vi "task_updateFirmware.vi"() -> ()   [LabVIEW 2015]
uses:
  Framework/pdbm_test_route/UsrDefine/TaskFeedbackCmd.ctl
  Framework/pdbm_test_route/UsrDefine/TaskReqst.ctl
  <vilib>/DAQmx/read.llb/DAQmx Read (Analog Wfm 1Chan NSamp).vi
  <vilib>/Utility/file.llb/Write Delimited Spreadsheet (string).vi
  <vilib>/measure/matone.llb/Extract Multiple Tone Information 1 Chan.vi
  <vilib>/DAQmx/miscellaneous.llb/DAQmx Fill In Error Info.vi
  <vilib>/measure/madcrms.llb/Basic Averaged DC-RMS for 1 Chan.vi
  <vilib>/measure/matone.llb/Extract Single Tone Information 1 Chan.vi
  Framework/pdbm_tasks/pdbm_tasks.lvlib
  <vilib>/measure/NI_MAPro.lvlib
  <vilib>/measure/NI_MABase.lvlib
  Framework/pdbm_test_route/pdbm_task_route.lvlib
panel:
  in  "uA_bank0":dbl=1.5 format="%#_13g"
  out "Sample rate":dbl=20000.0 format="%#_13g"
  out "Ver":string
  out "Task out":refnum<k21>="Stop"
  in  "Tab Control":enum32{"Current Tracking", "Image", "CSV LOG"}(tab)
  out "uA_bank1":dbl
  in  "Calib":bool
  in  "Power ON/OFF":bool
  in  "Profile":enum16{"SAM", "DIANA", "Other..."}(ring)
  in  "Take Picture":bool
  in  "Orginal":bool
  in  "Clear Graph":bool
  out "Amp(Vdc)":dbl
  out "Freq(Hz)":dbl
  out "Waveform Graph 3":waveform(dbl)(graph)
  in  "ZOOM M1M2":bool
  in  "ZOOM -":bool
  in  "ZOOM +":bool
  in  "stop":bool
  out "VDUT- Vbat":dbl
  in  "Acquire Mode":enum16{"Streaming", "Read All", "Stop"}(ring)
  in  "Measure":bool
  in  "Current Range":T1(ring)
  out "Source":dbl
  in  "USB":tag="Dev1"
  out "Min value":dbl
  out "Max value":dbl
  out "Delta(s)":sgl
  in  "Center":bool
  out "Average":dbl
  in  "mA/uA":bool
  out "Waveform_main":waveform(sgl)(graph)
  out "Waveform_sub":waveform(dbl)(graph)
  out "Average (uA)":dbl
  in  "DUT Voltage Selector":enum16{"3.8VDC", "2.9VDC", "3.7VDC", "4.0VDC"}(ring)=enum."2.9VDC"
  in  "file List":i32(listbox)
  out "2D Picture":picture
  out "uA 2":dbl format="%#_4g"
  out "Vbat":dbl format="%#_4g"
  out "current time":timestamp
  in  "Record uA & Vbat":bool
  in  "Path":path
  out "uA":dbl(graph)
  out "Vbat Monitor":dbl(graph)
  out "error out":errorcluster
  out "seconds since 1Jan1904":timestamp
  out "new_ver":string caption="New Version :"
  out "curr_version":string caption="Current Version :"
  out "Clear":bool=TRUE
  in  "error in (no error)":errorcluster
  in  "pdbm_task_data":T2
  # "Current"
  # "Voltage"
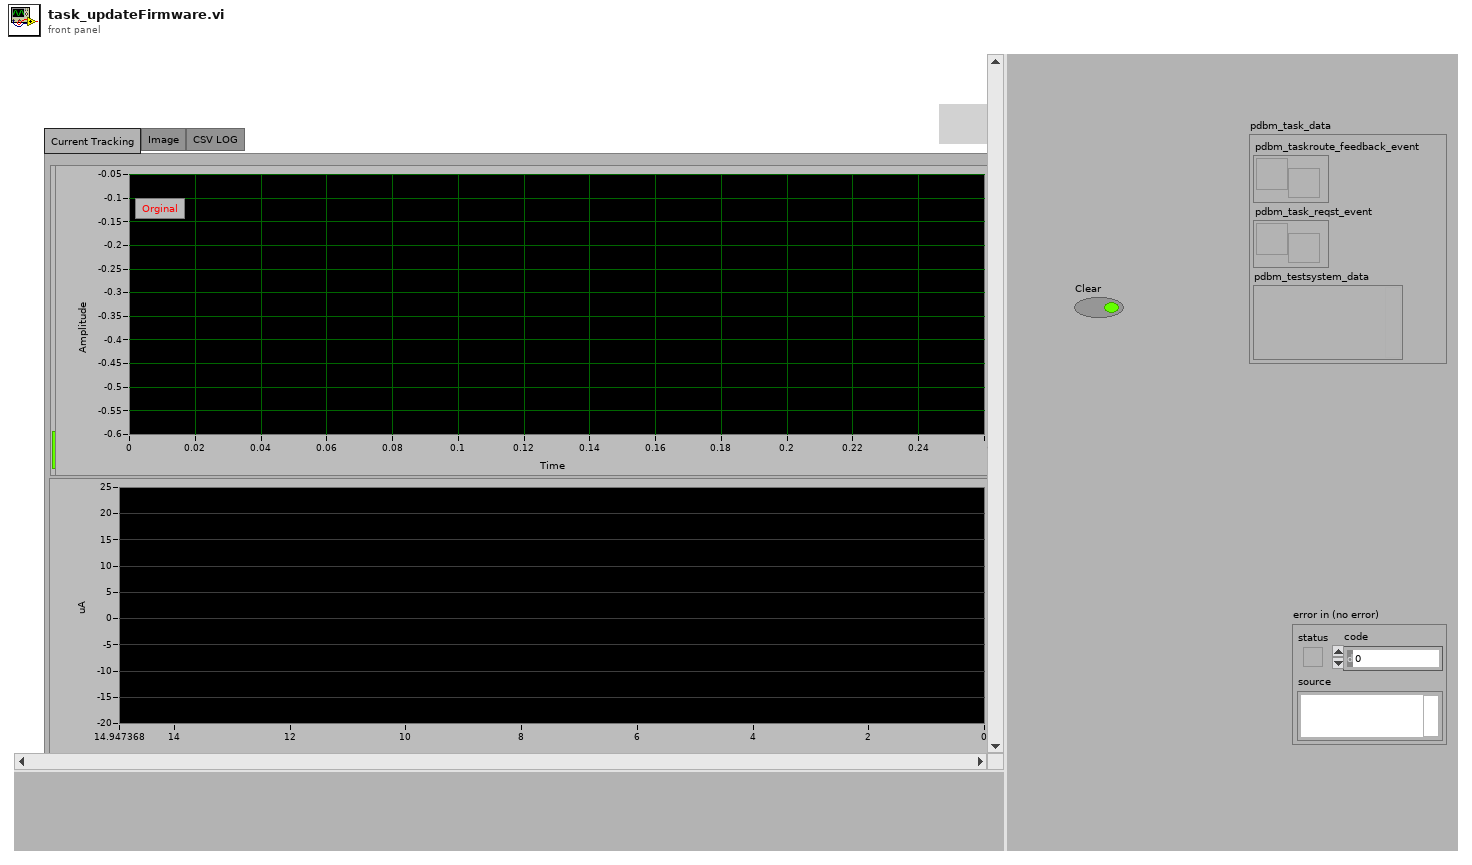
[diagram p1: front panel]
types:
  T1 = enum16{"Set uA Range ", "Set mA Range", "Measure Voltage"}
  T2 = cluster{"pdbm_taskroute_feedback_event":refnum<user-event>, "pdbm_task_reqst_event":refnum<user-event>, "pdbm_testsystem_data":variant}
  T3 = typedef "pdbm_tasks.lvlib/PDBM_TestSystem_Data.ctl" = cluster{"pdbm_general_report_info":refnum<vi>, "pdbm_task_progress":refnum<vi>, "pdbm_TestButton":refnum<vi>}
  T4 = cluster{"pdbm_task_reqst_event":refnum<user-event>, "pdbm_taskroute_feedback_event":refnum<user-event>}
  T5 = typedef "LVCursorListTypeDef.ctl" = cluster{"Name":string, "Color":u32, "Style":u8, "Point Style":u8, "Name Visible":bool, "Allow Drag":bool, "Cursor Mode":u32, "Plot":i32, "Index":i32, "Position":cluster{"X":dbl, "Y":dbl}, "X Scale":u32, "Y Scale":u32, "Watch Plots":i32[], "Watch All Plots":bool, "Plot Area":i32, "Label Offset":cluster{"X":dbl, "Y":dbl}}[]
  T6 = typedef "imagedata.ctl" = cluster{"image type":i32, "image depth":i32, "image":u8[], "mask":u8[], "colors":u32[], "Rectangle":cluster{"left":i16, "top":i16, "right":i16, "bottom":i16}}
  T7 = enum32{"none", "input signal", "detected signal", "residual signal"}
  T8 = cluster{"detected frequency":dbl, "detected amplitude":dbl, "detected phase (deg)":dbl}[]
  T9 = cluster{"detected frequency":dbl, "detected amplitude":dbl, "detected phase (deg)":dbl}
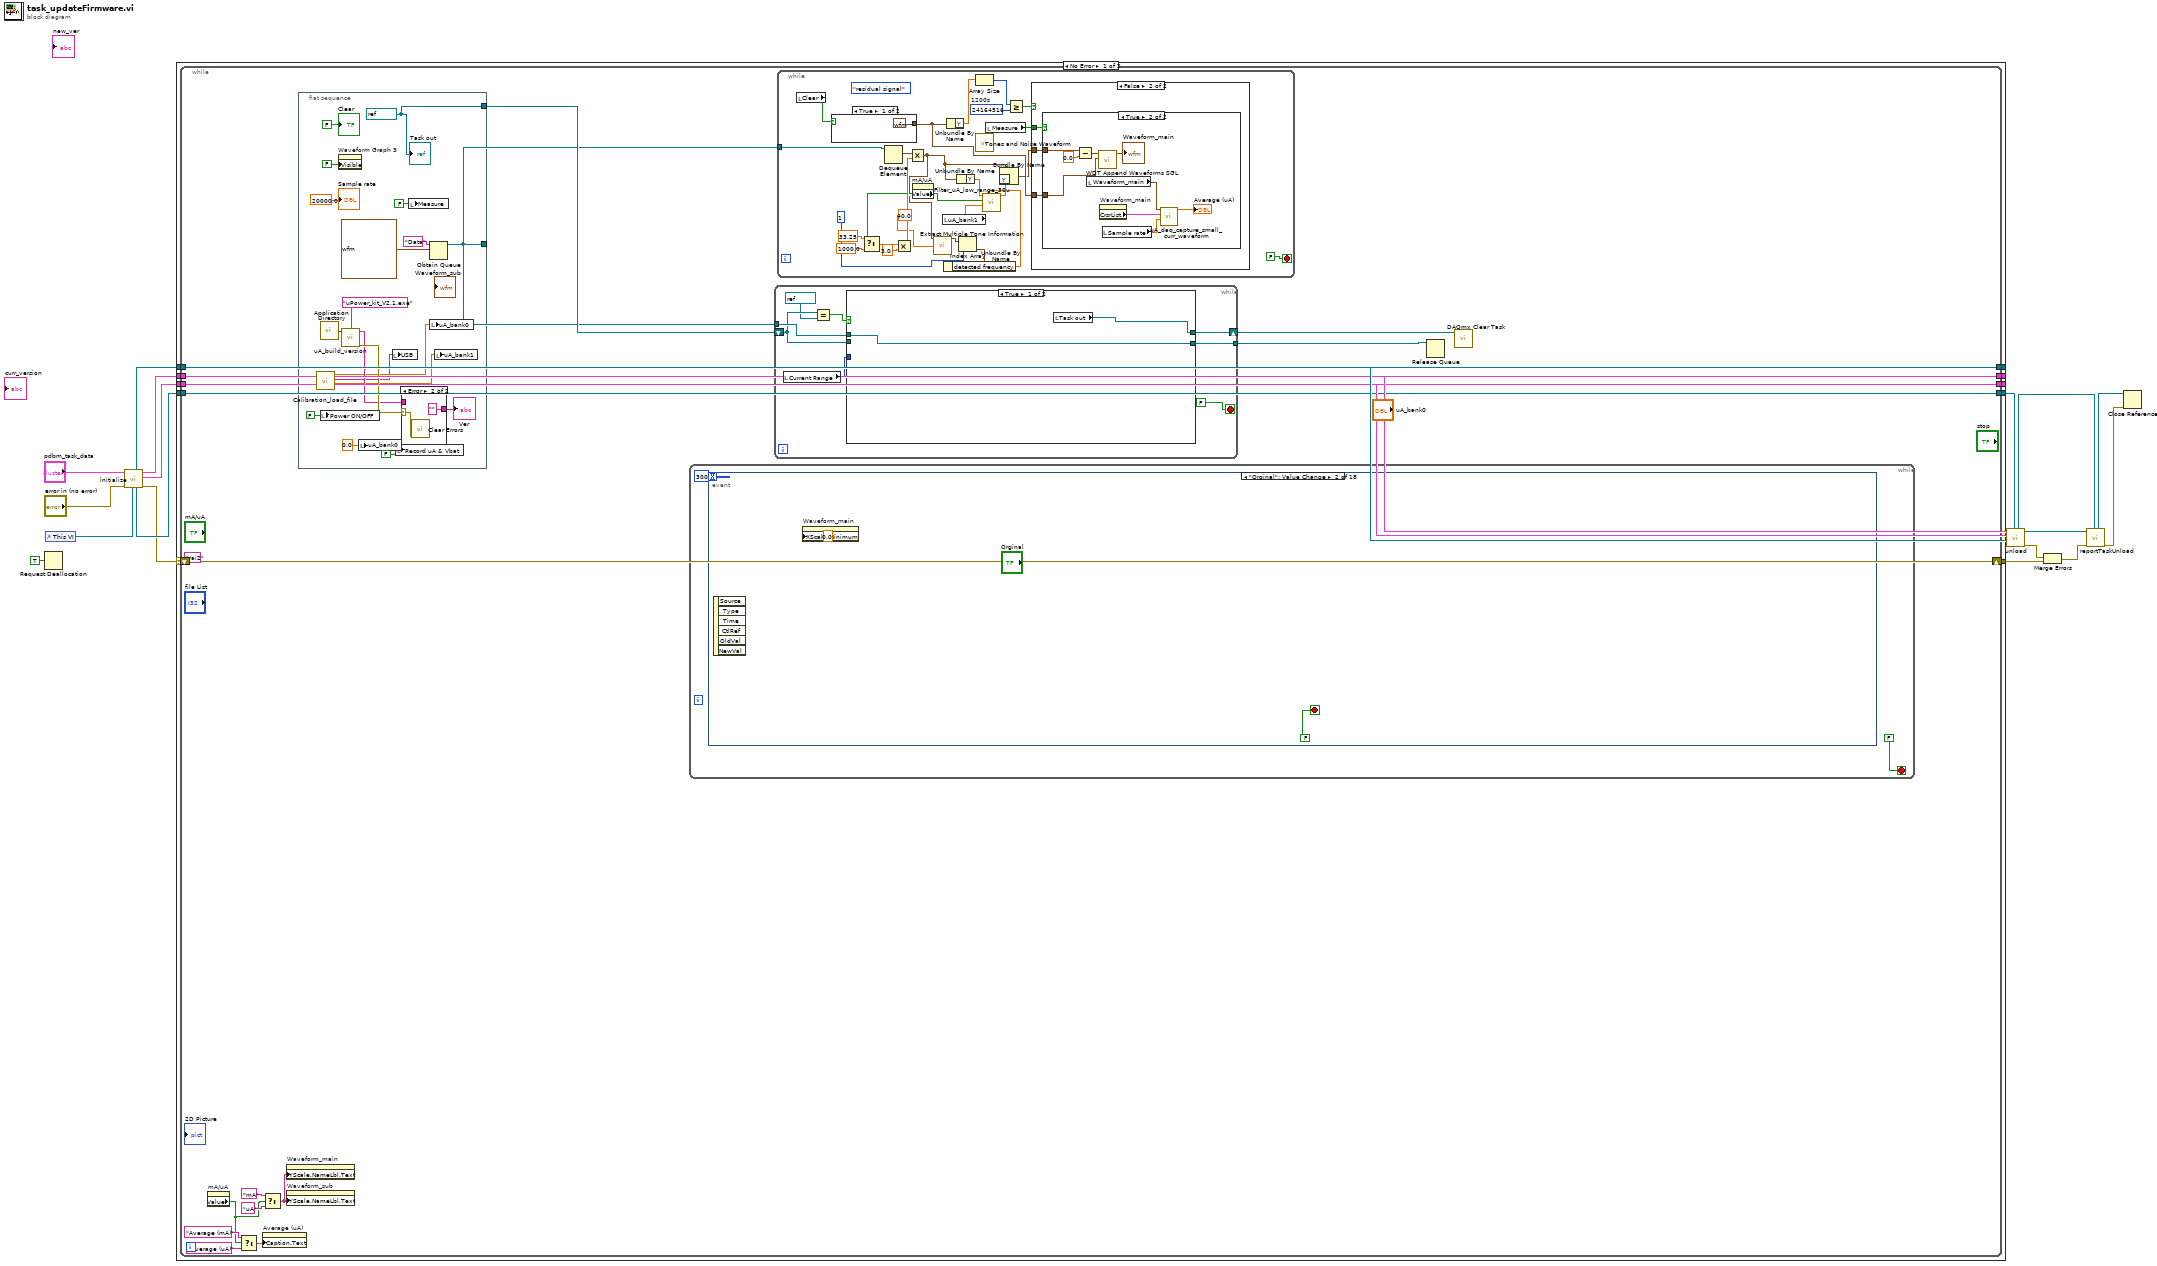
[diagram p0: block diagram]
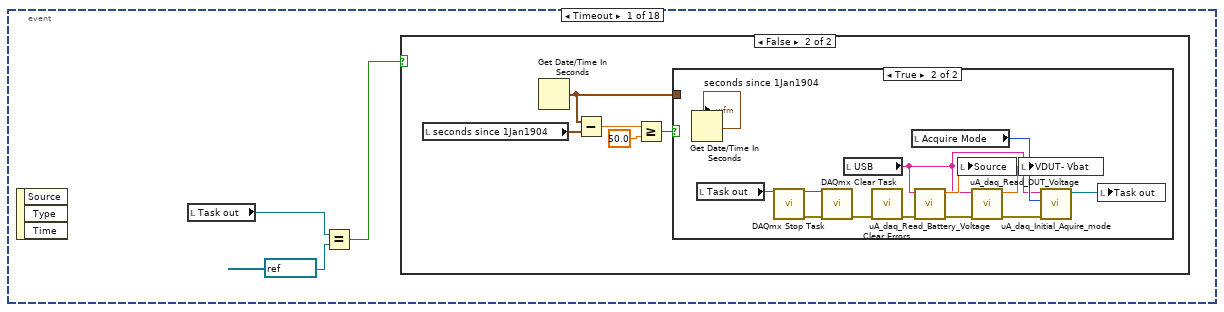
[diagram p3: hidden frame]
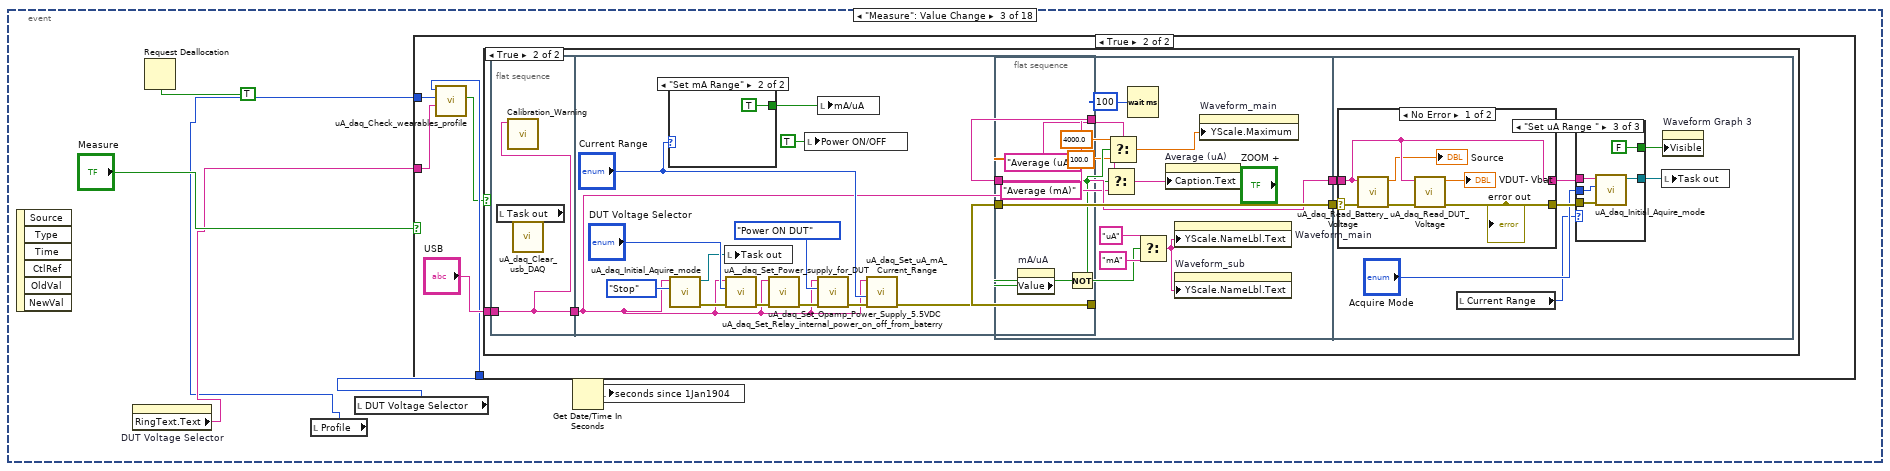
[diagram p6: hidden frame]
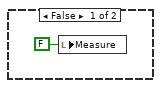
[diagram p8: hidden frame]
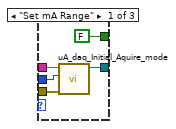
[diagram p9: hidden frame]
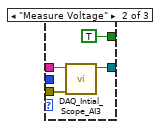
[diagram p10: hidden frame]
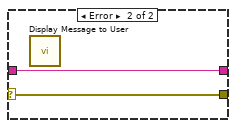
[diagram p11: hidden frame]
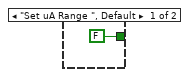
[diagram p12: hidden frame]
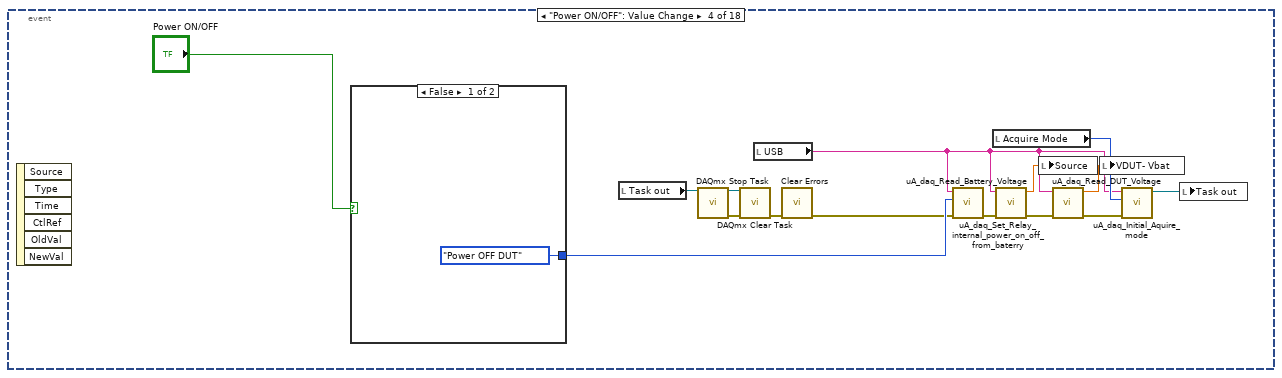
[diagram p13: hidden frame]
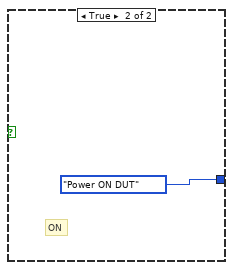
[diagram p14: hidden frame]
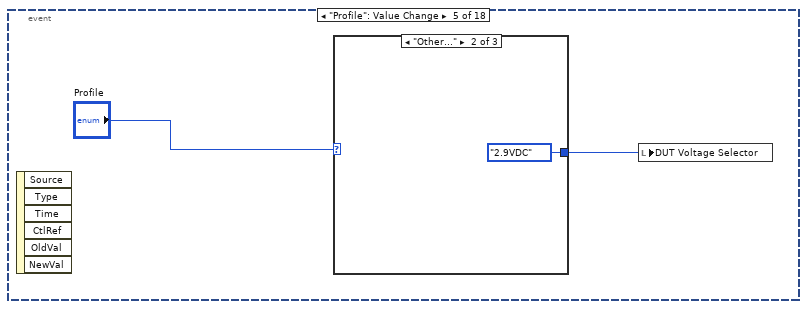
[diagram p15: hidden frame]
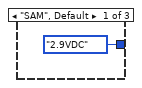
[diagram p16: hidden frame]
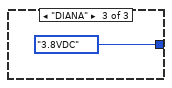
[diagram p17: hidden frame]
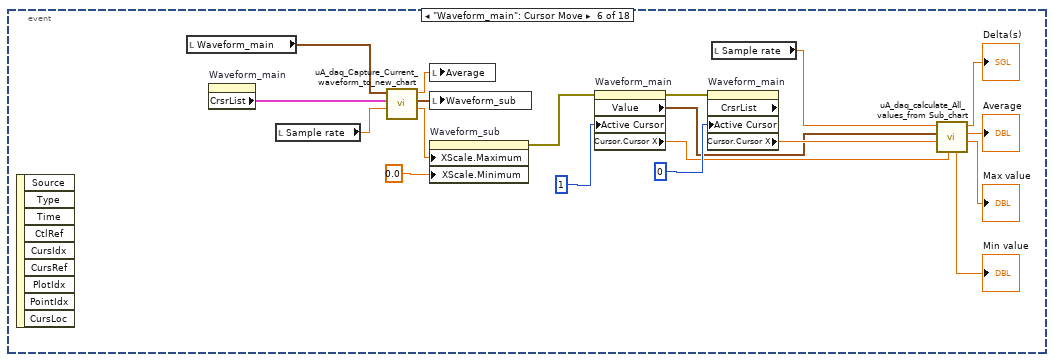
[diagram p18: hidden frame]
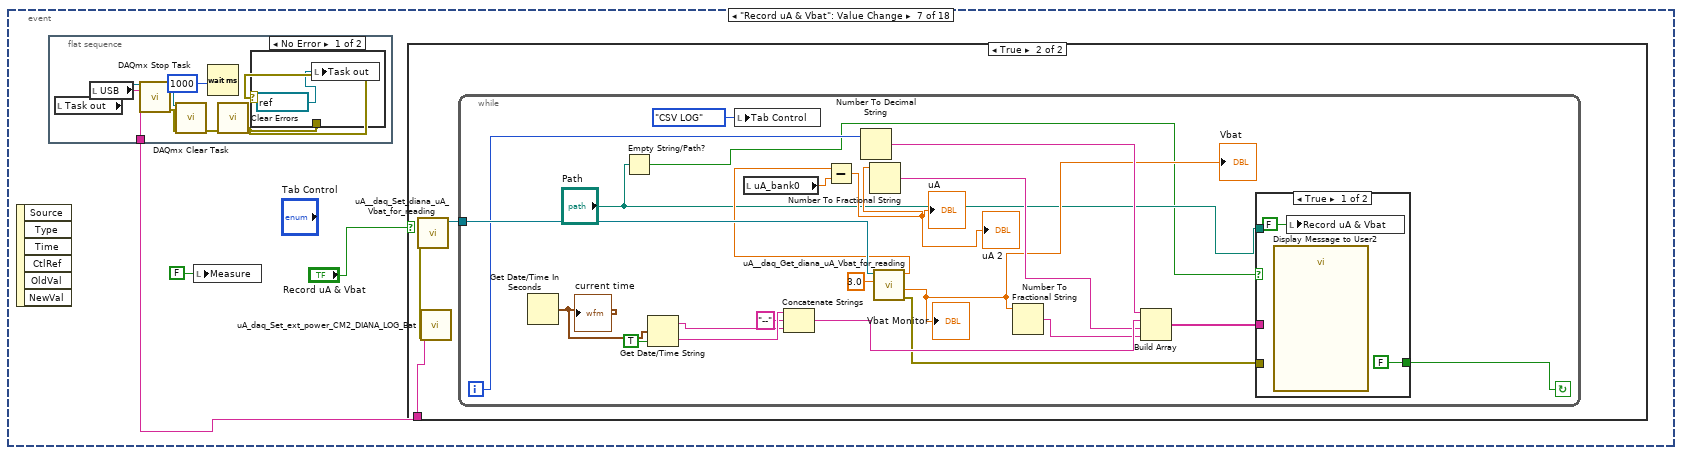
[diagram p19: hidden frame]
diagram:
  n1 = Request Deallocation(TRUE ("flag")) -> ()
  n2 = control-ref of="This VI"() -> (w19:refnum<vi>)
  n3 = call "initialize.vi"("TaskRef in"=w19, "error in"="error in (no error)", "pdbm_task_data"="pdbm_task_data") -> ("error out"=w15:errorcluster, "pdbm_task_data"=w3:T3, "pdbm_task_event"=w16:T4, "TaskRef out"=w17:refnum<vi>, "pdbm_task_reg_reqst_event"=w14:refnum<event-registration>)  [unwired: 4 in]
  n4 = case shown="No Error" w15 {
    selector: w15 -> [w29 w454]
    tunnel: w3 -> [w27 w452]
    tunnel: [w28 w454] -> w10
    tunnel: w17 -> [w22 w451]
    tunnel: w16 -> [w26 w453]
    tunnel: w14 -> [w30 w450]
    tunnel: [w25 w453] -> w13
    tunnel: [w24 w452] -> w12
    tunnel: [w23 w451] -> w2
    tunnel: [w21 w450] -> w11
    frame No Error {
      n5 = while {
        tunnel: w30 -> [w44]
        shift-right: [w43] -> w28
        shift-left: w29 -> [w43]
        tunnel: w22 -> [w45]
        tunnel: w27 -> [w46]
        tunnel: w26 -> [w47]
        tunnel: [w47] -> w25
        tunnel: [w46] -> w24
        tunnel: [w45] -> w23
        tunnel: [w44] -> w21
        stop <- FALSE ("stop") stop-if-true
        (unwired) "/ai2" ("string")
        n6 = property on="mA/uA" class="Bool (strict)"() -> ("Value"=w36:bool)  [unwired: 2 in, 2 out]
        n7 = Select(t="Average (mA)" ("Caption.Text"), s=w36, f="Average (uA)" ("Caption.Text")) -> (s? t:f=w34:string)
        n8 = property on="Average (uA)" class="DigNum (strict)"("Caption.Text"=w34) -> ()  [unwired: 2 in, 2 out]
        n9 = Select(t="mA" ("Caption.Text"), s=w36, f="uA" ("Caption.Text")) -> (s? t:f=w35:string)
        n10 = property on="Waveform_main" class="WFGraph (strict)"("YScale.NameLbl.Text"=w35) -> ()  [unwired: 2 in, 2 out]
        n11 = property on="Waveform_sub" class="WFGraph (strict)"("YScale.NameLbl.Text"=w35) -> ()  [unwired: 2 in, 2 out]
        n12 = flat-sequence {
          tunnel: [w58] -> w32
          tunnel: [w61] -> w31
          frame #0 {
            w58 = refnum<k21> "Stop" ("task out")
            n13 = call "Calibration_load_file.vi"() -> ("uABank1"=w51:dbl, "USB_DEV"=w50:string, "uABank0"=w52:dbl)  [unwired: 9 in]
            n14 = call <vilib>:"Application Directory.vi"() -> ("Application Directory"=w60:path)
            n15 = local write "Power ON/OFF"(FALSE ("Power ON/OFF")) -> ()
            n16 = property on="Waveform Graph 3" class="WFGraph (strict)"("Visible"=FALSE) -> ()  [unwired: 2 in, 2 out]
            n17 = call "uA_build_version.vi"("name or relative path"="uPower_kit_V2.1.exe", "path"=w60) -> ("error out"=w57:errorcluster, "FileVersion"=w56:string)  [unwired: 7 in, 1 out]
            n18 = local write "uA_bank0"(0.0 ("uA_calib_0")) -> ()
            n19 = local write "USB"(w50) -> ()
            n20 = local write "Record uA & Vbat"(FALSE ("Record uA & Vbat")) -> ()
            n21 = case shown="Error" w57 {
              selector: w57 -> [_ w69]
              tunnel: w56 -> [w67 _]
              tunnel: [w67 "" ("FileVersion")] -> w55
              frame No Error {
              }
              frame Error {
                n22 = call <vilib>:"Clear Errors.vi"("error in (no error)"=w69) -> ()  [unwired: 5 in, 2 out]
              }
            }
            "Ver" <- w55
            n23 = local write "Measure"(FALSE ("Measure")) -> ()
            n24 = Obtain Queue(name (unnamed)="Data", element data type=waveform(sgl) {"t0"=timestamp(0 s since 1904-01-01), "dt"=1.0, "Y"=[]} ("Waveform Chart 2")) -> (queue out=w61:refnum<queue>)  [unwired: 3 in, 2 out]
            n25 = local write "uA_bank0"(w52) -> ()
            n26 = local write "uA_bank1"(w51) -> ()
            "Clear" <- FALSE ("Clear")
            "Sample rate" <- 20000.0 ("Sample rate")
            "Task out" <- w58
          }
        }
        n27 = while {
          stop <- FALSE stop-if-true
          n28 = event shown="[1] \"Orginal\": Value Change" {
            selector: _ -> [_ _ _ _ _ _ _ _ _ _ _ _ _ _ _ _ _ _]
            dyn-events: _ -> [_ _ _ _ _ _ _ _ _ _ _ _ _ _ _ _ _ _]
            timeout: 300 -> [_ _ _ _ _ _ _ _ _ _ _ _ _ _ _ _ _ _]
            event Timeout {
              n29 = event-data() -> ()  [unwired: 1 in, 3 out]
              n30 = local read "Task out"() -> (w72:refnum<k21>)
              n31 = Equal?(x=w72, y=refnum<k21> "Stop") -> (x = y?=w73:bool)
              n32 = case shown="False" w73 {
                frame True {
                }
                frame False {
                  n33 = local read "seconds since 1Jan1904"() -> (w75:timestamp)
                  n34 = Get Date/Time In Seconds() -> (seconds since 1Jan1904=w76:timestamp)
                  n35 = Subtract(x=w76, y=w75) -> (x-y=w79:dbl)
                  n36 = Greater Or Equal?(x=w79, y=50.0) -> (x >= y?=w77:bool)
                  n37 = case shown="True" w77 {
                    tunnel: w76 -> [_ _]
                    frame False {
                    }
                    frame True {
                      n38 = Get Date/Time In Seconds() -> (seconds since 1Jan1904=→"seconds since 1Jan1904":timestamp)
                      n39 = local read "Task out"() -> (w89:refnum<k21>)
                      n40 = call <vilib>:"DAQmx Stop Task.vi"("task/channels in"=w89) -> ("task out"=w88:refnum<k21>, "error out"=w91:errorcluster)  [unwired: 13 in]
                      n41 = call <vilib>:"DAQmx Clear Task.vi"("task in"=w88, "error in"=w91) -> ("error out"=w90:errorcluster)  [unwired: 13 in]
                      n42 = local read "USB"() -> (w82:tag)
                      n43 = call <vilib>:"Clear Errors.vi"("error in (no error)"=w90) -> ("error out"=w87:errorcluster)  [unwired: 5 in, 1 out]
                      n44 = local read "Acquire Mode"() -> (w83:enum16{"Streaming", "Read All", "Stop"})
                      n45 = call "uA_daq_Read_Battery_Voltage.vi"("error in"=w87, "USB DAQ"=w82) -> ("error out"=w84:errorcluster, "Battery_Voltage"=w86:dbl)  [unwired: 8 in]
                      n46 = local write "Source"(w86) -> ()
                      n47 = call "uA_daq_Read_DUT_Voltage.vi"("error in"=w84, "USB DAQ"=w82) -> ("error out"=w81:errorcluster, "DUT_Voltage"=w85:dbl)  [unwired: 8 in]
                      n48 = local write "VDUT- Vbat"(w85) -> ()
                      n49 = call "uA_daq_Initial_Aquire_mode.vi"("error in"=w81, "Acquire Mode"=w83, "USB DAQ"=w82) -> ("Refnum out"=w80:refnum<k21>)  [unwired: 7 in, 1 out]
                      n50 = local write "Task out"(w80) -> ()
                    }
                  }
                }
              }
            }
            event "Orginal": Value Change {
              n51 = event-data() -> ()  [unwired: 1 in, 6 out]
              n52 = property on="Waveform_main" class="WFGraph (strict)"("XScale.Minimum"=0.0 ("X Scale.Range:Minimum")) -> ()  [unwired: 2 in, 2 out]
            }
            event "Measure": Value Change {
              n53 = event-data() -> ()  [unwired: 1 in, 6 out]
              n54 = property on="DUT Voltage Selector" class="Enum (strict)"() -> ("RingText.Text"=w96:string)  [unwired: 2 in, 2 out]
              n55 = Request Deallocation(TRUE ("flag")) -> ()
              n56 = local read "Profile"() -> (w94:enum16{"SAM", "DIANA", "Other..."})
              n57 = local read "DUT Voltage Selector"() -> (w95:enum16{"3.8VDC", "2.9VDC", "3.7VDC", "4.0VDC"})
              n58 = case shown="True" "Measure" {
                tunnel: w96 -> [_ w103]
                tunnel: w95 -> [_ w102]
                tunnel: w94 -> [_ w101]
                frame False {
                }
                frame True {
                  n59 = call "uA_daq_Check_wearables_profile.vi"("VDUT"=w103, "Profile"=w101, "DUT Voltage Selector"=w102) -> ("Profile"=w100:bool)  [unwired: 7 in, 1 out]
                  n60 = case shown="True" w100 {
                    tunnel: "USB" -> [_ w107]
                    frame False {
                      n61 = local write "Measure"(FALSE ("Measure")) -> ()
                    }
                    frame True {
                      n62 = flat-sequence {
                        tunnel: w107 -> [w156]
                        tunnel: [w156] -> w111
                        tunnel: [w165] -> w108
                        tunnel: [w159] -> w106
                        tunnel: w111 -> [w159]
                        frame #0 {
                          n63 = local read "Task out"() -> (w157:refnum<k21>)
                          n64 = call "Calibration_Warning.vi"("USB"=w156) -> ()  [unwired: 11 in]
                          n65 = call "uA_daq_Clear_usb_DAQ.vi"("Refnum in"=w157) -> ()  [unwired: 11 in]
                        }
                        frame #1 {
                          n66 = case shown="\"Set mA Range\"" "Current Range" {
                            tunnel: [FALSE ("mA/uA") TRUE ("mA/uA")] -> w163
                            frame "Set uA Range ", Default {
                            }
                            frame "Set mA Range" {
                            }
                          }
                          n67 = call "uA_daq_Initial_Aquire_mode.vi"("Acquire Mode"=enum16{"Streaming", "Read All", "Stop"}."Stop", "USB DAQ"=w159) -> ("error out"=w160:errorcluster, "Refnum out"=w161:refnum<k21>)  [unwired: 8 in]
                          n68 = local write "Task out"(w161) -> ()
                          n69 = call "uA__daq_Set_Power_supply_for_DUT.vi"("error in"=w160, "DUT Voltage Selector"="DUT Voltage Selector", "USB DAQ"=w159) -> ("error out"=w169:errorcluster)  [unwired: 8 in]
                          n70 = call "uA_daq_Set_Opamp_Power_Supply_5.5VDC.vi"("error in"=w169, "USB DAQ"=w159) -> ("error out"=w167:errorcluster)  [unwired: 9 in]
                          n71 = local write "Power ON/OFF"(TRUE ("Power ON/OFF")) -> ()
                          n72 = local write "mA/uA"(w163) -> ()
                          n73 = call "uA_daq_Set_Relay_internal_power_on_off_from_baterry.vi"("error in"=w167, "Power ON/OFF DUT"=enum16{"Power ON DUT", "Power OFF DUT"}."Power ON DUT", "USB DAQ"=w159) -> ("error out"=w166:errorcluster)  [unwired: 8 in]
                          n74 = call "uA_daq_Set_uA_mA_Current_Range.vi"("error in"=w166, "Current Range"="Current Range", "device name"=w159) -> ("error out"=w165:errorcluster)  [unwired: 8 in]
                        }
                      }
                      n75 = flat-sequence {
                        tunnel: w106 -> [w124]
                        tunnel: w108 -> [w125]
                        tunnel: [w125] -> w110
                        tunnel: [w124] -> w109
                        tunnel: w110 -> [w133]
                        tunnel: w109 -> [w132]
                        frame #0 {
                          n76 = property on="mA/uA" class="Bool (strict)"() -> ("Value"=w116:bool)  [unwired: 2 in, 2 out]
                          n77 = Not(x=w116) -> (.not. x?=w115:bool)
                          n78 = Select(t="Average (uA)" ("Caption.Text"), s=w115, f="Average (mA)" ("Caption.Text")) -> (s? t:f=w122:string)
                          n79 = Select(t=4000.0, s=w115, f=100.0) -> (s? t:f=w114:dbl)
                          n80 = Wait (ms)(milliseconds to wait=u32 100) -> ()  [unwired: 1 out]
                          n81 = Select(t="uA" ("Caption.Text"), s=w115, f="mA" ("Caption.Text")) -> (s? t:f=w117:string)
                          n82 = property on="Average (uA)" class="DigNum (strict)"("Caption.Text"=w122) -> ()  [unwired: 2 in, 2 out]
                          n83 = property on="Waveform_main" class="WFGraph (strict)"("YScale.NameLbl.Text"=w117) -> ()  [unwired: 2 in, 2 out]
                          n84 = property on="Waveform_sub" class="WFGraph (strict)"("YScale.NameLbl.Text"=w117) -> ()  [unwired: 2 in, 2 out]
                          n85 = property on="Waveform_main" class="WFGraph (strict)"("YScale.Maximum"=w114) -> ()  [unwired: 2 in, 2 out]
                        }
                        frame #1 {
                          n86 = case shown="No Error" w133 {
                            selector: w133 -> [w151 w155]
                            tunnel: w132 -> [w149 w154]
                            tunnel: [w150 w155] -> w131
                            tunnel: [w149 w154] -> w130
                            frame No Error {
                              n87 = call "uA_daq_Read_Battery_Voltage.vi"("error in"=w151, "USB DAQ"=w149) -> ("error out"=w153:errorcluster, "Battery_Voltage"=→"Source":dbl)  [unwired: 8 in]
                              n88 = call "uA_daq_Read_DUT_Voltage.vi"("error in"=w153, "USB DAQ"=w149) -> ("error out"=w150:errorcluster, "DUT_Voltage"=→"VDUT- Vbat":dbl)  [unwired: 8 in]
                              "error out" <- w150
                            }
                            frame Error {
                              n89 = call "Display Message to User"() -> ()  [unwired: 10 in, 2 out]
                            }
                          }
                          n90 = local read "Current Range"() -> (w127:T1)
                          n91 = case shown="\"Set uA Range \"" w127 {
                            tunnel: w131 -> [w138 w140 w147]
                            tunnel: w130 -> [w137 w142 w146]
                            tunnel: [w136 w141 w145] -> w129
                            tunnel: "Acquire Mode" -> [w135 _ w144]
                            tunnel: [FALSE ("Visible") TRUE ("Visible") FALSE ("Visible")] -> w126
                            frame "Set mA Range" {
                              n92 = call "uA_daq_Initial_Aquire_mode.vi"("error in"=w138, "Acquire Mode"=w135, "USB DAQ"=w137) -> ("Refnum out"=w136:refnum<k21>)  [unwired: 7 in, 1 out]
                            }
                            frame "Measure Voltage" {
                              n93 = call "DAQ_Intial_Scope_AI3.vi"("error in"=w140, "physical channel"=w142) -> ("task out"=w141:refnum<k21>)  [unwired: 8 in, 1 out]
                            }
                            frame "Set uA Range " {
                              n94 = call "uA_daq_Initial_Aquire_mode.vi"("error in"=w147, "Acquire Mode"=w144, "USB DAQ"=w146) -> ("Refnum out"=w145:refnum<k21>)  [unwired: 7 in, 1 out]
                            }
                          }
                          n95 = local write "Task out"(w129) -> ()
                          n96 = property on="Waveform Graph 3" class="WFGraph (strict)"("Visible"=w126) -> ()  [unwired: 2 in, 2 out]
                        }
                      }
                    }
                  }
                }
              }
              n97 = Get Date/Time In Seconds() -> (seconds since 1Jan1904=w98:timestamp)
              n98 = local write "seconds since 1Jan1904"(w98) -> ()
            }
            event "Power ON/OFF": Value Change {
              n99 = event-data() -> ()  [unwired: 1 in, 6 out]
              n100 = case shown="False" "Power ON/OFF" {
                tunnel: [enum16{"Power ON DUT", "Power OFF DUT"}."Power OFF DUT" ("Power ON/OFF DUT") enum16{"Power ON DUT", "Power OFF DUT"}."Power ON DUT" ("Power ON/OFF DUT")] -> w177
                frame False {
                }
                frame True {
                  # "ON"
                }
              }
              n101 = local read "Task out"() -> (w185:refnum<k21>)
              n102 = call <vilib>:"DAQmx Stop Task.vi"("task/channels in"=w185) -> ("task out"=w184:refnum<k21>, "error out"=w187:errorcluster)  [unwired: 13 in]
              n103 = call <vilib>:"DAQmx Clear Task.vi"("task in"=w184, "error in"=w187) -> ("error out"=w186:errorcluster)  [unwired: 13 in]
              n104 = local read "USB"() -> (w176:tag)
              n105 = call <vilib>:"Clear Errors.vi"("error in (no error)"=w186) -> ("error out"=w175:errorcluster)  [unwired: 5 in, 1 out]
              n106 = call "uA_daq_Set_Relay_internal_power_on_off_from_baterry.vi"("error in"=w175, "Power ON/OFF DUT"=w177, "USB DAQ"=w176) -> ("error out"=w174:errorcluster)  [unwired: 8 in]
              n107 = local read "Acquire Mode"() -> (w181:enum16{"Streaming", "Read All", "Stop"})
              n108 = call "uA_daq_Read_Battery_Voltage.vi"("error in"=w174, "USB DAQ"=w176) -> ("error out"=w173:errorcluster, "Battery_Voltage"=w183:dbl)  [unwired: 8 in]
              n109 = local write "Source"(w183) -> ()
              n110 = call "uA_daq_Read_DUT_Voltage.vi"("error in"=w173, "USB DAQ"=w176) -> ("error out"=w180:errorcluster, "DUT_Voltage"=w182:dbl)  [unwired: 8 in]
              n111 = local write "VDUT- Vbat"(w182) -> ()
              n112 = call "uA_daq_Initial_Aquire_mode.vi"("error in"=w180, "Acquire Mode"=w181, "USB DAQ"=w176) -> ("Refnum out"=w179:refnum<k21>)  [unwired: 7 in, 1 out]
              n113 = local write "Task out"(w179) -> ()
            }
            event "Profile": Value Change {
              n114 = event-data() -> ()  [unwired: 1 in, 6 out]
              n115 = case shown="\"Other...\"" "Profile" {
                tunnel: [enum16{"3.8VDC", "2.9VDC", "3.7VDC", "4.0VDC"}."2.9VDC" ("DUT Voltage Selector") enum16{"3.8VDC", "2.9VDC", "3.7VDC", "4.0VDC"}."2.9VDC" ("DUT Voltage Selector") enum16{"3.8VDC", "2.9VDC", "3.7VDC", "4.0VDC"}."3.8VDC" ("DUT Voltage Selector")] -> w190
                frame "SAM", Default {
                }
                frame "Other..." {
                }
                frame "DIANA" {
                }
              }
              n116 = local write "DUT Voltage Selector"(w190) -> ()
            }
            event "Waveform_main": Cursor Move {
              n117 = event-data() -> ()  [unwired: 1 in, 9 out]
              n118 = local read "Waveform_main"() -> (w203:waveform(sgl))
              n119 = property on="Waveform_main" class="WFGraph (strict)"() -> ("CrsrList"=w213:T5)  [unwired: 2 in, 2 out]
              n120 = local read "Sample rate"() -> (w202:dbl)
              n121 = call "uA_daq_Capture_Current_waveform_to_new_chart.vi"("Sample rate"=w202, "CrsrList"=w213, "Waveform_main"=w203) -> ("Numeric"=w210:dbl, "Waveform"=w211:waveform(sgl), "Numeric 2"=w212:sgl)  [unwired: 6 in]
              n122 = local write "Average"(w212) -> ()
              n123 = local write "Waveform_sub"(w211) -> ()
              n124 = property on="Waveform_sub" class="WFGraph (strict)"("XScale.Maximum"=w210, "XScale.Minimum"=0.0 ("X Scale.Range:Minimum")) -> (error out=w195:errorcluster)  [unwired: 2 in, 1 out]
              n125 = property on="Waveform_main" class="WFGraph (strict)"(error in=w195, "Active Cursor"=u32 1) -> (error out=w205:errorcluster, "Value"=w204:waveform(sgl), "Cursor.Cursor X"=w207:dbl)  [unwired: 1 in, 1 out]
              n126 = property on="Waveform_main" class="WFGraph (strict)" props=["CrsrList", "Active Cursor", "Cursor", "Cursor X"](error in=w205, "Active Cursor"=u32 0) -> ("Cursor.Cursor X"=w206:dbl)  [unwired: 1 in, 3 out]
              n127 = local read "Sample rate"() -> (w201:dbl)
              n128 = call "uA_daq_calculate_All_values_from Sub_chart.vi"("Cursor.Cursor X 2"=w207, "Cursor.Cursor X"=w206, "Value"=w204, "Sample rate"=w201) -> ("Max value"=→"Max value":dbl, "Average"=→"Average":dbl, "Delta(s)"=→"Delta(s)":sgl, "Min value"=→"Min value":dbl)  [unwired: 4 in]
            }
            event "Record uA & Vbat": Value Change {
              n129 = event-data() -> ()  [unwired: 1 in, 6 out]
              n130 = flat-sequence {
                tunnel: [w223] -> w215
                frame #0 {
                  n131 = local read "Task out"() -> (w219:refnum<k21>)
                  n132 = local read "USB"() -> (w223:tag)
                  n133 = call <vilib>:"DAQmx Stop Task.vi"("task/channels in"=w219) -> ("task out"=w218:refnum<k21>, "error out"=w221:errorcluster)  [unwired: 13 in]
                  n134 = call <vilib>:"DAQmx Clear Task.vi"("task in"=w218, "error in"=w221) -> ("error out"=w220:errorcluster)  [unwired: 13 in]
                  n135 = Wait (ms)(milliseconds to wait=u32 1000) -> ()  [unwired: 1 out]
                  n136 = call <vilib>:"Clear Errors.vi"("error in (no error)"=w220) -> ("error out"=w217:errorcluster)  [unwired: 5 in, 1 out]
                  n137 = case shown="No Error" w217 {
                    tunnel: w217 -> [_ _]
                    frame No Error {
                      n138 = local write "Task out"(refnum<k21> "Stop" ("y")) -> ()
                    }
                    frame Error {
                    }
                  }
                }
              }
              n139 = local write "Measure"(FALSE ("Measure")) -> ()
              n140 = case shown="True" "Record uA & Vbat" {
                tunnel: w215 -> [_ w227]
                frame False {
                }
                frame True {
                  n141 = call "uA_daq_Set_ext_power_CM2_DIANA_LOG_Bat.vi"("USB DAQ in"=w227) -> ("error out"=w228:errorcluster, "USB DAQ out"=w226:tag)  [unwired: 9 in]
                  n142 = call "uA__daq_Set_diana_uA_Vbat_for_reading.vi"("error in (no error)"=w228, "USB DAQ in"=w226) -> ("Refnum out"=w225:refnum<k21>)  [unwired: 8 in, 1 out]
                  n143 = while {
                    tunnel: w225 -> [w250]
                    i -> [w240]
                    stop <- w229 continue-if-true
                    n144 = Get Date/Time In Seconds() -> (seconds since 1Jan1904=w249:timestamp)
                    "current time" <- w249
                    n145 = Empty String/Path?(string/path="Path") -> (empty?=w230:bool)
                    n146 = Get Date/Time String(seconds (now)=w249, want seconds? (F)=TRUE) -> (date string=w247:string, time string=w248:string)  [unwired: 1 in]
                    n147 = local write "Tab Control"(enum32{"Current Tracking", "Image", "CSV LOG"}."CSV LOG" ("Tab Control")) -> ()
                    n148 = local read "uA_bank0"() -> (w235:dbl)
                    n149 = Concatenate Strings(w248, "--" ("string"), w247) -> (w245:string)
                    n150 = Number To Decimal String(number=w240) -> (decimal integer string=w239:string)  [unwired: 1 in]
                    n151 = call "uA__daq_Get_diana_uA_Vbat_for_reading.vi"("Coef"=3.0, "Refnum in"=w250) -> ("error out"=w236:errorcluster, "Vbat"=w238:dbl, "uA Current"=w234:dbl)  [unwired: 5 in, 2 out]
                    "Vbat Monitor" <- w238
                    "Vbat" <- w238
                    n152 = Subtract(x=w234, y=w235) -> (x-y=w233:dbl)
                    "uA" <- w233
                    "uA 2" <- w233
                    n153 = Number To Fractional String(number=w233) -> (F-format string=w244:string)  [unwired: 3 in]
                    n154 = Number To Fractional String(number=w238) -> (F-format string=w243:string)  [unwired: 3 in]
                    n155 = Build Array(w239, w245, w244, w243) -> (w242:string[])
                    n156 = case shown="True" w230 {
                      tunnel: w242 -> [_ w256]
                      tunnel: w236 -> [_ w255]
                      tunnel: "Path" -> [_ w254]
                      tunnel: [FALSE ("Record uA & Vbat") w253] -> w229
                      frame True {
                        n157 = call "Display Message to User2"() -> ()  [unwired: 10 in, 2 out]
                        n158 = local write "Record uA & Vbat"(FALSE ("Record uA & Vbat")) -> ()
                      }
                      frame False {
                        n159 = local read "Record uA & Vbat"() -> (w253:bool)
                        n160 = case shown="No Error" w255 {
                          tunnel: w256 -> [w260 _]
                          tunnel: w254 -> [w257 _]
                          frame No Error {
                            n161 = call-poly <vilib>:"Write Delimited Spreadsheet.vi"("file path (dialog if empty)"=w257, "1D data"=w260, "append to file? (F)"=TRUE, "delimiter (\\t)"=";" ("delimiter (\\t)")) -> ()  [unwired: 10 in, 2 out]
                          }
                          frame Error {
                          }
                        }
                      }
                    }
                  }
                }
              }
            }
            event "Calib": Value Change {
              n162 = event-data() -> ()  [unwired: 1 in, 6 out]
              n163 = property on="mA/uA" class="Bool (strict)"() -> ("Value"=w263:bool)  [unwired: 2 in, 2 out]
              n164 = case shown="False" w263 {
                tunnel: [w264 _] -> w261
                frame False {
                  w271 = 3.0  # Coef 10Ohm:3
                  # "uA"
                  n165 = flat-sequence {
                    tunnel: [w280] -> w269
                    frame #0 {
                      n166 = call "Display Message to User3"() -> ()  [unwired: 10 in, 2 out]
                      n167 = local write "Measure"(FALSE ("Measure")) -> ()
                    }
                    frame #1 {
                      n168 = local read "Task out"() -> (w277:refnum<k21>)
                      n169 = Wait (ms)(milliseconds to wait=u32 1000) -> ()  [unwired: 1 out]
                      n170 = call <vilib>:"DAQmx Stop Task.vi"("task/channels in"=w277) -> ("task out"=w276:refnum<k21>, "error out"=w278:errorcluster)  [unwired: 13 in]
                      n171 = call <vilib>:"DAQmx Clear Task.vi"("task in"=w276, "error in"=w278) -> ("error out"=w275:errorcluster)  [unwired: 13 in]
                      n172 = case shown="No Error" w275 {
                        frame No Error {
                          n173 = local write "Task out"(refnum<k21> "Stop" ("y")) -> ()
                        }
                        frame Error {
                        }
                      }
                      n174 = local read "USB"() -> (w280:tag)
                    }
                  }
                  n175 = call "uA_daq_Set_ext_power_CM2_DIANA_LOG_Bat.vi"("USB DAQ in"=w269) -> ("error out"=w266:errorcluster, "USB DAQ out"=w273:tag)  [unwired: 9 in]
                  n176 = call "uA__daq_Set_diana_uA_Vbat_for_reading.vi"("error in (no error)"=w266, "USB DAQ in"=w273) -> ("error out"=w267:errorcluster, "Refnum out"=w272:refnum<k21>)  [unwired: 8 in]
                  n177 = call "uA__daq_Get_diana_uA_Vbat_for_reading.vi"("error in (no error)"=w267, "Coef"=w271, "Refnum in"=w272) -> ("error out"=w268:errorcluster, "uA Current"=w270:dbl)  [unwired: 4 in, 3 out]
                  n178 = local write "uA_bank0"(w270) -> ()
                  n179 = call "Calibration_Read_streaming_3s.vi"("error in (no error)"=w268, "USB"=w269) -> ("error out"=w264:errorcluster, "uABank1"=w265:dbl)  [unwired: 8 in]
                  "uA_bank1" <- w265
                  n180 = call "Calibration_Save_file.vi"("USB_DEV"=w269, "uABank1"=w265, "uABank0"=w270) -> ()  [unwired: 9 in]
                }
                frame True {
                  # "mA"
                }
              }
              n181 = call "Display Message to User4"("error in (no error)"=w261, "Enable"=TRUE) -> ()  [unwired: 8 in, 2 out]
            }
            event "Clear Graph": Value Change {
              n182 = event-data() -> ()  [unwired: 1 in, 6 out]
              n183 = flat-sequence {
                frame #0 {
                  w282 = waveform(sgl) {"t0"=timestamp(0 s since 1904-01-01), "dt"=1.0, "Y"=[]} ("Waveform_main")
                  n184 = local write "Waveform_main"(w282) -> ()
                  n185 = local write "Clear"(TRUE ("Clear")) -> ()
                  n186 = Wait (ms)(milliseconds to wait=u32 500) -> ()  [unwired: 1 out]
                  n187 = local write "Waveform_sub"(w282) -> ()
                }
                frame #1 {
                  n188 = local write "Clear"(FALSE ("Clear")) -> ()
                }
              }
            }
            event "ZOOM +": Value Change {
              n189 = event-data() -> ()  [unwired: 1 in, 6 out]
              n190 = property on="Waveform_main" class="WFGraph (strict)" props=["XScale", "Range", "XScale", "Increment", "XScale", "Maximum", "XScale", "Minimum"]() -> ("XScale.Maximum"=w291:dbl, "XScale.Minimum"=w287:dbl)  [unwired: 2 in, 4 out]
              n191 = Subtract(x=w291, y=0.1) -> (x-y=w289:dbl)
              n192 = Add(x=w287, y=0.1) -> (x+y=w286:dbl)
              n193 = property on="Waveform_main" class="WFGraph (strict)"("XScale.Maximum"=w289, "XScale.Minimum"=w286) -> ()  [unwired: 2 in, 2 out]
            }
            event "ZOOM -": Value Change {
              n194 = event-data() -> ()  [unwired: 1 in, 6 out]
              n195 = property on="Waveform_main" class="WFGraph (strict)" props=["XScale", "Range", "XScale", "Increment", "XScale", "Maximum", "XScale", "Minimum"]() -> ("XScale.Maximum"=w300:dbl, "XScale.Minimum"=w296:dbl)  [unwired: 2 in, 4 out]
              n196 = Subtract(x=w296, y=0.1) -> (x-y=w293:dbl)
              n197 = Less Than 0?(x=w293) -> (x < 0?=w295:bool)
              n198 = Add(x=w300, y=0.1) -> (x+y=w298:dbl)
              n199 = Select(t=0.0, s=w295, f=w293) -> (s? t:f=w292:dbl)
              n200 = property on="Waveform_main" class="WFGraph (strict)"("XScale.Maximum"=w298, "XScale.Minimum"=w292) -> ()  [unwired: 2 in, 2 out]
            }
            event "ZOOM M1M2": Value Change {
              n201 = event-data() -> ()  [unwired: 1 in, 6 out]
              n202 = property on="Waveform_main" class="WFGraph (strict)"("Active Cursor"=u32 0) -> (error out=w307:errorcluster)  [unwired: 2 in, 1 out]
              n203 = property on="Waveform_main" class="WFGraph (strict)"(error in=w307) -> (error out=w304:errorcluster, "Cursor.Cursor X"=w302:dbl)  [unwired: 1 in, 1 out]
              n204 = property on="Waveform_main" class="WFGraph (strict)"(error in=w304, "Active Cursor"=u32 1) -> (error out=w306:errorcluster)  [unwired: 1 in, 1 out]
              n205 = property on="Waveform_main" class="WFGraph (strict)"(error in=w306) -> ("Cursor.Cursor X"=w301:dbl)  [unwired: 1 in, 2 out]
              n206 = Greater?(x=w302, y=w301) -> (0:w303:bool)
              n207 = case shown="True" w303 {
                tunnel: w302 -> [w310 w312]
                tunnel: w301 -> [w309 w311]
                frame False {
                  n208 = property on="Waveform_main" class="WFGraph (strict)"("XScale.Maximum"=w309, "XScale.Minimum"=w310) -> ()  [unwired: 2 in, 2 out]
                }
                frame True {
                  n209 = property on="Waveform_main" class="WFGraph (strict)"("XScale.Maximum"=w312, "XScale.Minimum"=w311) -> ()  [unwired: 2 in, 2 out]
                }
              }
            }
            event "Waveform_main": Mouse Down {
              n210 = event-data() -> ()  [unwired: 1 in, 8 out]
            }
            event "Tab Control": Value Change {
              n211 = event-data() -> ()  [unwired: 1 in, 6 out]
              n212 = call <vilib>:"Application Directory.vi"() -> ("Application Directory"=w315:path)
              n213 = call <userlib>:"List Directory__ogtk.vi"("pattern"="*.bmp", "directory path"=w315) -> ("file names"=w313:string[])  [unwired: 2 in, 3 out]
              n214 = property on="file List" class="LstBox (strict)"("Item Names"=w313) -> ()  [unwired: 2 in, 2 out]
            }
            event "Center": Value Change {
              n215 = event-data() -> ()  [unwired: 1 in, 6 out]
              n216 = property on="Waveform_main" class="WFGraph (strict)"() -> ("XScale.Maximum"=w320:dbl, "XScale.Minimum"=w319:dbl)  [unwired: 2 in, 2 out]
              n217 = Add(x=w320, y=w319) -> (x+y=w318:dbl)
              n218 = Divide(x=w318, y=2.0) -> (x/y=w316:dbl)
              n219 = property on="Waveform_main" class="WFGraph (strict)" props=["Value", "Active Cursor", "Cursor", "Cursor X"]("Active Cursor"=u32 1, "Cursor.Cursor X"=w316) -> (error out=w321:errorcluster)  [unwired: 2 in, 2 out]
              n220 = property on="Waveform_main" class="WFGraph (strict)" props=["CrsrList", "Active Cursor", "Cursor", "Cursor X"](error in=w321, "Active Cursor"=u32 0, "Cursor.Cursor X"=w316) -> ()  [unwired: 1 in, 3 out]
            }
            event "stop": Value Change {
              n221 = event-data() -> ()  [unwired: 1 in, 6 out]
              n222 = flat-sequence {
                frame #0 {
                  n223 = local read "Task out"() -> (w325:refnum<k21>)
                  n224 = call <vilib>:"DAQmx Stop Task.vi"("task/channels in"=w325) -> ("task out"=w324:refnum<k21>, "error out"=w327:errorcluster)  [unwired: 13 in]
                  n225 = call <vilib>:"DAQmx Clear Task.vi"("task in"=w324, "error in"=w327) -> ("error out"=w326:errorcluster)  [unwired: 13 in]
                  n226 = call <vilib>:"Clear Errors.vi"("error in (no error)"=w326) -> ()  [unwired: 5 in, 2 out]
                }
                frame #1 {
                  n227 = local read "USB"() -> (w331:tag)
                  n228 = call "uA_daq_Set_Relay_internal_power_on_off_from_baterry.vi"("Power ON/OFF DUT"=enum16{"Power ON DUT", "Power OFF DUT"}."Power OFF DUT", "USB DAQ"=w331) -> ("error out"=w330:errorcluster)  [unwired: 9 in]
                  n229 = call "uA_daq_Set_Opamp_Power_Supply_Zero_voltageVDC.vi"("error in"=w330, "USB DAQ"=w331) -> ("error out"=w328:errorcluster)  [unwired: 9 in]
                  n230 = call <vilib>:"Clear Errors.vi"("error in (no error)"=w328) -> ()  [unwired: 5 in, 2 out]
                }
                frame #2 {
                  n231 = local read "Ver"() -> (w332:string)
                  n232 = Empty String/Path?(string/path=w332) -> (empty?=w333:bool)
                  n233 = case shown="True" w333 {
                    frame True {
                    }
                    frame False {
                      n234 = Quit LabVIEW(quit? (T)=TRUE) -> ()
                    }
                  }
                }
                frame #3 {
                  n235 = Stop(stop? (T)=TRUE) -> ()
                }
              }
            }
            event "file List": Value Change {
              n236 = event-data() -> ()  [unwired: 1 in, 6 out]
              n237 = property on="file List" class="LstBox (strict)"() -> ("Value"=w342:i32, "Item Names"=w343:string[])  [unwired: 2 in, 2 out]
              n238 = Index Array(array=w343, index=w342) -> (element=w338:string)
              n239 = call <vilib>:"Application Directory.vi"() -> ("Application Directory"=w339:path)
              n240 = Build Path(base path=w339, name or relative path=w338) -> (appended path=w337:path)
              n241 = call <vilib>:"Read BMP File.vi"("path to BMP file"=w337) -> ("image data"=w341:T6)  [unwired: 8 in, 2 out]
              n242 = call <vilib>:"Draw Flattened Pixmap.vi"("image data"=w341) -> ("new picture"=w340:picture)  [unwired: 8 in]
              n243 = property on="2D Picture" class="Pict"("Value"=w340, "ZoomFactor"=sgl 0.75 ("Zoom Factor")) -> ()  [unwired: 2 in, 2 out]
            }
            event "Take Picture": Value Change {
              n244 = event-data() -> ()  [unwired: 1 in, 6 out]
              n245 = call <vilib>:"Application Directory.vi"() -> ("Application Directory"=w345:path)
              n246 = call "File Dialog"("start path"=w345, "pattern (all files)"="*.bmp", "pattern label"="*.bmp") -> ("selected path"=w351:path, "error out"=w348:errorcluster)  [unwired: 9 in, 2 out]
              n247 = control-ref of="This VI"() -> (w349:refnum<vi>)
              n248 = invoke on="Invoke Node" class="VI" method="FP.Get Image"(reference=w349, "image depth"=enum32{"File", "Clipboard"}."File" ("Target")) -> ("image data"=w350:T6)  [unwired: 4 in, 5 out]
              n249 = call <vilib>:"Clear Errors.vi"("error in (no error)"=w348) -> ()  [unwired: 5 in, 2 out]
              n250 = call <vilib>:"Write BMP File.vi"("image data"=w350, "path to BMP file"=w351) -> ()  [unwired: 8 in, 2 out]
            }
          }
        }
        n251 = while {
          tunnel: w31 -> [w400]
          tunnel: [w399] -> w41
          shift-right: [w395] -> w33
          shift-left: w32 -> [w397]
          stop <- FALSE ("stop (F)") stop-if-true
          n252 = local read "Current Range"() -> (w394:T1)
          n253 = Equal?(x=w397, y=refnum<k21> "Stop") -> (x = y?=w393:bool)
          n254 = case shown="True" w393 {
            tunnel: w400 -> [w402 w407]
            tunnel: [w402 w406] -> w399
            tunnel: w397 -> [_ w405]
            tunnel: [w401 w404] -> w395
            tunnel: w394 -> [_ w403]
            frame True {
              n255 = local read "Task out"() -> (w401:refnum<k21>)
            }
            frame False {
              n256 = case shown="\"Set uA Range \"" w403 {
                tunnel: w407 -> [w418 w423 w445]
                tunnel: [w417 w423 w444] -> w406
                tunnel: w405 -> [w416 w434 w443]
                tunnel: [w415 w433 w442] -> w404
                frame "Set mA Range" {
                  w414 = 10.0  # timeout (s)
                  n257 = call-poly <vilib>:"DAQmx Read.vi"("task/channels in"=w416, "number of samples per channel"=10000, "timeout"=w414) -> ("data"=w409:waveform(dbl), "error out"=w412:errorcluster)  [unwired: 10 in, 1 out]
                  n258 = Unbundle By Name(w409) -> ("Y"=w411:dbl[])
                  n259 = Reverse 1D Array(array=w411) -> (reversed array=w408:dbl[])
                  n260 = Bundle By Name(cluster=w409, "Y"=w408) -> (w410:waveform(dbl))
                  n261 = case shown="No Error" w412 {
                    selector: w412 -> [_ w422]
                    tunnel: w418 -> [w421 _]
                    tunnel: [w420 _] -> w417
                    tunnel: w410 -> [w419 _]
                    frame No Error {
                      n262 = Enqueue Element(queue=w421, element=w419) -> (queue out=w420:refnum<queue>)  [unwired: 2 in, 2 out]
                    }
                    frame Error {
                      n263 = call <vilib>:"Clear Errors.vi"("error in (no error)"=w422) -> ()  [unwired: 5 in, 2 out]
                    }
                  }
                  n264 = local read "Task out"() -> (w415:refnum<k21>)
                }
                frame "Measure Voltage" {
                  w432 = 10.0  # timeout (s)
                  n265 = call-poly <vilib>:"DAQmx Read.vi"("task/channels in"=w434, "number of samples per channel"=5000, "timeout"=w432) -> ("data"=w427:waveform(dbl), "error out"=w430:errorcluster)  [unwired: 10 in, 1 out]
                  "Waveform Graph 3" <- w427
                  n266 = call <vilib>:"Clear Errors.vi"("error in (no error)"=w430) -> ()  [unwired: 5 in, 2 out]
                  n267 = call-poly <vilib>:"Basic Averaged DC-RMS.vi"("averaging type"=enum16{"Linear", "Exponential"}."Linear", "signal in"=w427) -> ("error out"=w424:errorcluster, "DC value"=→"Amp(Vdc)":dbl)  [unwired: 6 in, 2 out]
                  n268 = call-poly <vilib>:"Extract Single Tone Information.vi"("time signal in"=w427) -> ("error out"=w428:errorcluster, "detected frequency"=→"Freq(Hz)":dbl)  [unwired: 5 in, 4 out]
                  n269 = local read "Task out"() -> (w433:refnum<k21>)
                  n270 = call <vilib>:"Clear Errors.vi"("error in (no error)"=w428) -> ()  [unwired: 5 in, 2 out]
                  n271 = call <vilib>:"Clear Errors.vi"("error in (no error)"=w424) -> ()  [unwired: 5 in, 2 out]
                }
                frame "Set uA Range " {
                  w441 = 10.0  # timeout (s)
                  n272 = call-poly <vilib>:"DAQmx Read.vi"("task/channels in"=w443, "number of samples per channel"=10000, "timeout"=w441) -> ("data"=w436:waveform(dbl), "error out"=w439:errorcluster)  [unwired: 10 in, 1 out]
                  n273 = Unbundle By Name(w436) -> ("Y"=w438:dbl[])
                  n274 = Reverse 1D Array(array=w438) -> (reversed array=w435:dbl[])
                  n275 = Bundle By Name(cluster=w436, "Y"=w435) -> (w437:waveform(dbl))
                  n276 = case shown="Error" w439 {
                    selector: w439 -> [_ w449]
                    tunnel: w445 -> [w448 _]
                    tunnel: [w447 _] -> w444
                    tunnel: w437 -> [w446 _]
                    frame No Error {
                      n277 = Enqueue Element(queue=w448, element=w446) -> (queue out=w447:refnum<queue>)  [unwired: 2 in, 2 out]
                    }
                    frame Error {
                      n278 = call <vilib>:"Clear Errors.vi"("error in (no error)"=w449) -> ()  [unwired: 5 in, 2 out]
                    }
                  }
                  n279 = local read "Task out"() -> (w442:refnum<k21>)
                }
              }
            }
          }
        }
        n280 = while {
          tunnel: w31 -> [w373]
          stop <- FALSE stop-if-true
          (unwired) T7."residual signal" ("export mode")
          w366 = 24164516  # 1200s
          n281 = local read "Clear"() -> (w371:bool)
          n282 = case shown="True" w371 {
            tunnel: [waveform(sgl) {"t0"=timestamp(0 s since 1904-01-01), "dt"=1.0, "Y"=[]} ("Waveform_main") w392] -> w370
            frame True {
            }
            frame False {
              n283 = local read "Waveform_main"() -> (w392:waveform(sgl))
            }
          }
          n284 = Dequeue Element(queue=w373) -> (element=w372:waveform(sgl))  [unwired: 2 in, 3 out]
          n285 = property on="mA/uA" class="Bool (strict)"() -> ("Value"=w359:bool)  [unwired: 2 in, 2 out]
          n286 = Select(t=sgl 33.25 ("y"), s=w359, f=sgl 1000.0 ("y")) -> (s? t:f=w365:sgl)
          n287 = Multiply(x=w365, y=sgl 3.0) -> (x*y=w364:sgl)
          n288 = Multiply(x=w372, y=w364) -> (x*y=w357:waveform(sgl))
          n289 = call-poly <vilib>:"Extract Multiple Tone Information.vi"("time signal in"=w357, "threshold"=40.0 ("Numeric 2")) -> ("multiple tone information"=w356:T8)  [unwired: 11 in, 2 out]
          n290 = local read "uA_bank1"() -> (w358:dbl)
          n291 = Unbundle By Name(w370) -> ("Y"=w369:sgl[])
          n292 = Unbundle By Name(w357) -> ("Y"=w361:sgl[])
          n293 = Index Array(array=w356, index=u16 1 ("Index")) -> (element=w355:T9)
          n294 = Unbundle By Name(w355) -> ("detected frequency"=w352:dbl)
          n295 = Array Size(array=w369) -> (size(s)=w376:i32)
          n296 = call <vilib>:"Tones and Noise Waveform.vi"() -> ()  [unwired: 10 in, 2 out]
          n297 = call "Filter_uA_low_range_30u.vi"("Frequency"=w352, "uA_calib_0"=w358, "mA/uA"=w359, "in"=w361) -> ("out"=w360:dbl[])  [unwired: 7 in]
          n298 = local read "Measure"() -> (w368:bool)
          n299 = Bundle By Name(cluster=w357, "Y"=w360) -> (w362:waveform(sgl))
          n300 = Greater Or Equal?(x=w376, y=w366) -> (x >= y?=w367:bool)
          n301 = case shown="False" w367 {
            tunnel: w362 -> [_ w381]
            tunnel: w370 -> [_ w380]
            tunnel: w368 -> [_ w379]
            frame True {
              n302 = local write "Measure"(FALSE ("Measure")) -> ()
            }
            frame False {
              n303 = case shown="True" w379 {
                tunnel: w381 -> [_ w389]
                tunnel: w380 -> [_ w382]
                frame False {
                }
                frame True {
                  n304 = Subtract(x=w389, y=sgl 0.0) -> (x-y=w383:waveform(sgl))
                  n305 = local read "Waveform_main"() -> (w386:waveform(sgl))
                  n306 = call "WDT Append Waveforms SGL.vi"("waveform B"=w382, "waveform A"=w383) -> ("waveform out"=→"Waveform_main":waveform(sgl))  [unwired: 8 in, 1 out]
                  n307 = property on="Waveform_main" class="WFGraph (strict)"() -> ("CrsrList"=w387:T5)  [unwired: 2 in, 2 out]
                  n308 = local read "Sample rate"() -> (w385:dbl)
                  n309 = call "uA_daq_capture_small_curr_waveform.vi"("Sample rate"=w385, "CrsrList"=w387, "Waveform_main"=w386) -> ("Numeric"=→"Average (uA)":sgl)  [unwired: 8 in]
                }
              }
            }
          }
        }
        n310 = Release Queue(queue=w41) -> ()  [unwired: 2 in, 3 out]
        n311 = call <vilib>:"DAQmx Clear Task.vi"("task in"=w33) -> ()  [unwired: 14 in, 1 out]
      }
    }
    frame Error {
    }
  }
  n312 = call "unload.vi"("TaskRef in"=w2, "pdbm_task_reg_reqst_event"=w11, "pdbm_task_data"=w12, "pdbm_task_event"=w13) -> ("error out"=w9:errorcluster, "pdbm_taskroute_feedback_event"=w8:refnum<user-event>, "TaskRef out"=w1:refnum<vi>)  [unwired: 5 in]
  n313 = Merge Errors(w9, w10) -> (w7:errorcluster)
  n314 = call "reportTaskUnload.vi"("TaskRef"=w1, "error in (no error)"=w7, "pdbm_taskroute_feedback_event"=w8) -> ("error out"=w4:errorcluster, "TaskRef out"=w5:refnum<vi>)  [unwired: 6 in, 1 out]
  n315 = Close Reference(reference=w5, error in (no error)=w4) -> ()  [unwired: 1 out]
